vi "chaosui-default-decode.vi"(8 "JSON string":string) -> (0 "parse_error":i32, 1 "dev_error":bool, 2 "dev_state":T1, 3 "timestamp":u64, 4 "dev_error_status":string)   [LabVIEW 2012]
uses:
  ChaosDevState.ctl
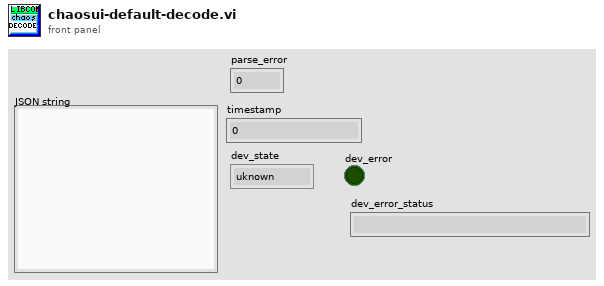
[diagram p1: front panel]
types:
  T1 = typedef "ChaosDevState.ctl" = enum16{"uknown", "stop", "init", "deinit", "start"}
  T2 = cluster{"error_status":string, "log_status":string, "dev_status":string}
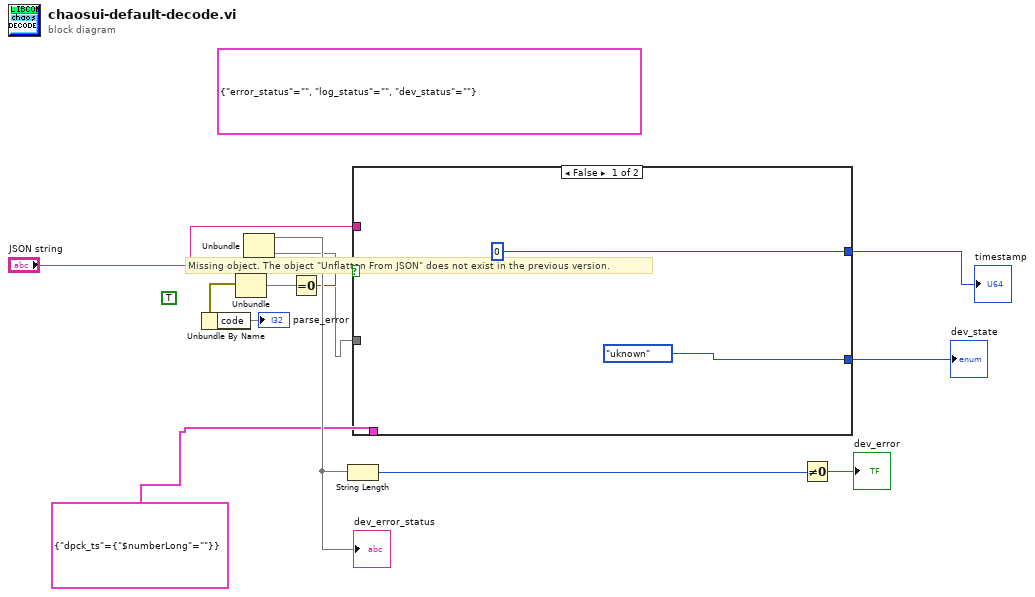
[diagram p0: block diagram]
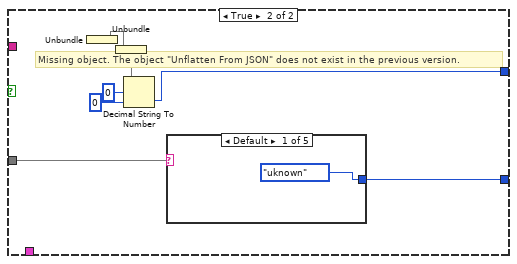
[diagram p2: hidden frame]
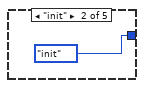
[diagram p3: hidden frame]
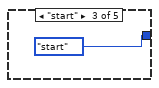
[diagram p4: hidden frame]
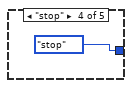
[diagram p5: hidden frame]
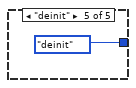
[diagram p6: hidden frame]
diagram:
  w8 = T2 {"error_status"="", "log_status"="", "dev_status"=""}
  (unwired) TRUE ("default null elements? (F)")
  # "Missing object. The object \"Unflatten From JSON\" does not exist in the previous version."
  n1 = Unbundle() -> (w12:errorcluster, "code"=w13)  [unwired: 2 out]
  n2 = Unbundle By Name(w12) -> ("code"=→"parse_error")
  n3 = Unbundle() -> ("error_status"=w7, "dev_status"=w2)  [unwired: 1 in, 1 out]
  "dev_error_status" <- w7
  n4 = Equal To 0?(x=w13) -> (x = 0?=w6:bool)
  n5 = String Length(string=w7) -> (length=w11:i32)
  n6 = case shown="False" w6 {
    tunnel: "JSON string" -> [_ _]
    tunnel: cluster{"dpck_ts":cluster{"$numberLong":string}} {"dpck_ts"={"$numberLong"=""}} -> [_ w23]
    tunnel: [u64 0 w19] -> w3
    tunnel: w2 -> [_ w17]
    tunnel: [ChaosDevState."uknown" ("dev_state") w16] -> w1
    frame False {
    }
    frame True {
      # "Missing object. The object \"Unflatten From JSON\" does not exist in the previous version."
      n7 = Unbundle() -> ("dpck_ts"=w22)  [unwired: 1 in]
      n8 = Unbundle(w22) -> (w18)
      n9 = Decimal String To Number(string=w18, offset=0, default (0L)=u64 0 ("default (0 I32)")) -> (number=w19:u64)  [unwired: 1 out]
      n10 = case shown="Default" w17 {
        tunnel: [ChaosDevState."uknown" ("dev_state") ChaosDevState."init" ("dev_state") ChaosDevState."start" ("dev_state") ChaosDevState."stop" ("dev_state") ChaosDevState."deinit" ("dev_state")] -> w16
        frame Default {
        }
        frame "init" {
        }
        frame "start" {
        }
        frame "stop" {
        }
        frame "deinit" {
        }
      }
    }
  }
  "timestamp" <- w3
  "dev_state" <- w1
  n11 = Not Equal To 0?(x=w11) -> (x != 0?=→"dev_error":bool)
